vi "Actor.vi"(4 "Creator":refnum<class "Msg Type Strategy.lvclass">, 6 "Creator Alias":string, 7 "jettl":refnum<class "jettl.lvclass">, 8 "Self Alias":string, 9 "Queue of Self":refnum<queue>, 10 "Msg Type Strategy":refnum<class "Msg Type Strategy.lvclass">) -> ()   [LabVIEW 2021, in "jettl.lvlib"]
uses:
  jettl.lvlib
  Base Queue/Base Queue/Base Queue.lvclass
  Addresses/Addresses.lvlib
  Last Ack Created Msg Strategy/Last Ack Created Msg Strategy.lvlib
  Last Ack Creator Msg Strategy/Last Ack Creator Msg Strategy.lvlib
  Msg Type Strategy/Msg Type Strategy/Msg Type Strategy.lvclass
  Queue/Queue.lvclass
  jettl/jettl.lvclass
  C:/git/jettl/jettl/jettl/jettl/jettl.lvclass
  C:/git/jettl/jettl/Merge Error Msg Strategy/Merge Error/Merge Error.lvclass
  C:/git/jettl/jettl/jettl/Queue/Queue.lvclass
  C:/git/jettl/jettl/Create Msg Strategy/Create/Create.lvclass
  C:/git/jettl/jettl/jettl/Last Ack Created Msg Strategy/Last Ack Created/Last Ack Created.lvclass
  C:/git/jettl/jettl/jettl/Last Ack Creator Msg Strategy/Last Ack Creator/Last Ack Creator.lvclass
  C:/git/jettl/jettl/Override Error Msg Strategy/Override Error/Override Error.lvclass
  C:/git/jettl/jettl/Setup Msg Strategy/Setup/Setup.lvclass
  C:/git/jettl/jettl/Teardown Msg Strategy/Teardown/Teardown.lvclass
  C:/git/jettl/jettl/jettl/Base Queue/Base Queue/Base Queue.lvclass
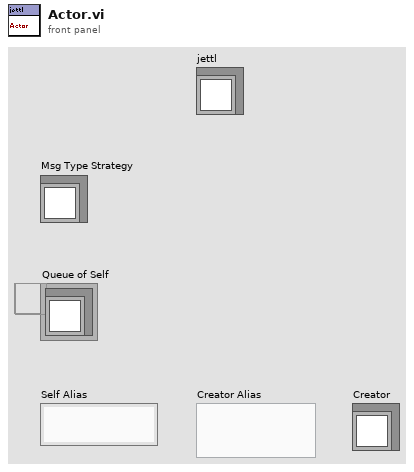
[diagram p1: front panel]
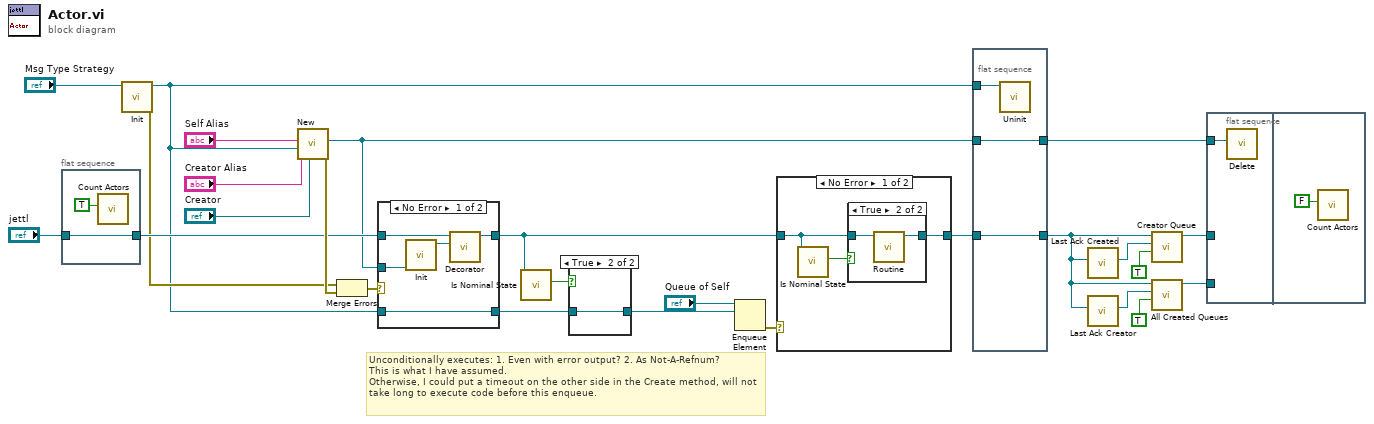
[diagram p0: block diagram]
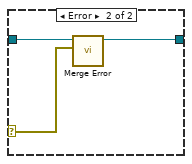
[diagram p3: hidden frame]
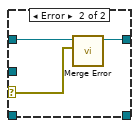
[diagram p5: hidden frame]
diagram:
  # "Unconditionally executes: 1. Even with error output? 2. As Not-A-Refnum?\nThis is what I have assumed.\nOtherwise, I could put a timeout on the other side in the Create method, will not take long to execute code before this enqueue."
  n1 = flat-sequence {
    tunnel: [w27] -> w24
    tunnel: "jettl" -> [w27]
    frame #0 {
      n2 = call "Count Actors.vi"("Increment?"=TRUE) -> ()  [unwired: 11 in]
    }
  }
  n3 = call-dynamic "Init.vi"("Msg Type Strategy in"="Msg Type Strategy") -> ("error out"=w6:errorcluster, "Msg Type Strategy out"=w5:refnum<class "Msg Type Strategy.lvclass">)  [unwired: 9 in]
  n4 = call "New.vi"("Creator"="Creator", "Creator Alias"="Creator Alias", "Self"=w5, "Self Alias"="Self Alias") -> ("error out"=w25:errorcluster, "Addresses DVR"=w22:refnum<data-value>)  [unwired: 6 in]
  n5 = Merge Errors(w6, w25) -> (w26:errorcluster)
  n6 = case shown="No Error" w26 {
    selector: w26 -> [_ w35]
    tunnel: [w31 w36] -> w10
    tunnel: w24 -> [w30 w34]
    tunnel: w5 -> [w33 _]
    tunnel: [w33 _] -> w12
    tunnel: w22 -> [w32 _]
    frame No Error {
      n7 = call "Init.vi"("Queue Mailbox"=w32) -> ("Base Queue out"=w29:refnum<class "Base Queue.lvclass">)  [unwired: 10 in]
      n8 = call-dynamic "Decorator.vi"("jettl"=w29, "jettl in"=w30) -> ("jettl out"=w31:refnum<class "jettl.lvclass">)  [unwired: 9 in]
    }
    frame Error {
      n9 = call-dynamic "Merge Error.vi"("Error"=w35, "Merge Error in"=w34) -> ("Merge Error out"=w36:refnum<class "jettl.lvclass">)  [unwired: 9 in]
    }
  }
  n10 = call-dynamic "Is Nominal State.vi"("jettl in"=w10) -> ("Is Nominal State?"=w11:bool)  [unwired: 10 in]
  n11 = case shown="True" w11 {
    tunnel: [_ w37] -> w13
    tunnel: w12 -> [_ w37]
    frame False {
    }
    frame True {
    }
  }
  n12 = Enqueue Element(queue="Queue of Self", element=w13) -> (error out=w9:errorcluster)  [unwired: 2 in, 2 out]
  n13 = case shown="No Error" w9 {
    selector: w9 -> [_ w44]
    tunnel: [w40 w45] -> w19
    tunnel: w10 -> [w38 w46]
    frame No Error {
      n14 = call-dynamic "Is Nominal State.vi"("jettl in"=w38) -> ("Is Nominal State?"=w39:bool)  [unwired: 10 in]
      n15 = case shown="True" w39 {
        tunnel: w38 -> [w41 w43]
        tunnel: [w41 w42] -> w40
        frame False {
        }
        frame True {
          n16 = call-dynamic "Routine.vi"("jettl in"=w43) -> ("jettl out"=w42:refnum<class "jettl.lvclass">)  [unwired: 10 in]
        }
      }
    }
    frame Error {
      n17 = call-dynamic "Merge Error.vi"("Error"=w44, "Merge Error in"=w46) -> ("Merge Error out"=w45:refnum<class "jettl.lvclass">)  [unwired: 9 in]
    }
  }
  n18 = flat-sequence {
    tunnel: w22 -> [w49]
    tunnel: w5 -> [w48]
    tunnel: w19 -> [w47]
    tunnel: [w47] -> w8
    tunnel: [w49] -> w16
    frame #0 {
      n19 = call-dynamic "Uninit.vi"("Msg Type Strategy in"=w48) -> ()  [unwired: 10 in, 1 out]
    }
  }
  n20 = call "Last Ack Created.vi"("jettl"=w8) -> ("Msg Strategy"=w21:refnum<class "Msg Strategy.lvclass">)  [unwired: 10 in]
  n21 = call "Last Ack Creator.vi"("jettl"=w8) -> ("Msg Strategy"=w20:refnum<class "Msg Strategy.lvclass">)  [unwired: 10 in]
  n22 = call-dynamic "Creator Queue.vi"("Priority?"=TRUE, "Msg Strategy"=w21, "Queue in"=w8) -> ("Queue out"=w14:refnum<class "Queue.lvclass">)  [unwired: 8 in]
  n23 = call-dynamic "All Created Queues.vi"("Priority?"=TRUE, "Msg Strategy"=w20, "Queue in"=w8) -> ("Queue out"=w15:refnum<class "Queue.lvclass">)  [unwired: 8 in]
  n24 = flat-sequence {
    tunnel: w16 -> [w50]
    tunnel: w14 -> [_]
    tunnel: w15 -> [_]
    frame #0 {
      n25 = call "Delete.vi"("Addresses DVR"=w50) -> ()  [unwired: 10 in, 1 out]
    }
    frame #1 {
      n26 = call "Count Actors.vi"("Increment?"=FALSE) -> ()  [unwired: 11 in]
    }
  }
